vi "URL to OS Path String.vi"(3 "URL Path String":string) -> (1 "OS Path String":string)   [LabVIEW 2020, in "GPack.lvlib" / "LVProject.lvclass"]
uses:
  LVProject.lvclass
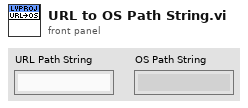
[diagram p1: front panel]
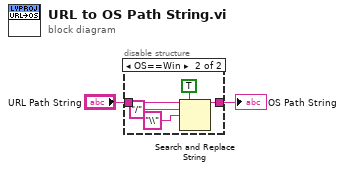
[diagram p0: block diagram]
diagram:
  n1 = disable-structure shown="OS==Win" {
    disable-tunnel: "URL Path String" -> [w3 w8]
    disable-tunnel: [w3 w4] -> w1
    frame condition #0 {
    }
    frame condition #1 (active) {
      n2 = Search and Replace String(replace all?=TRUE ("replace all? (F)"), input string=w8, search string="/", replace string="\\" ("search string")) -> (result string=w4:string)  [unwired: 4 in, 3 out]
    }
  }
  "OS Path String" <- w1
